vi "Write to IR DB.vi"(8 "error in (no error)":errorcluster, 9 "Values":u16[](array[numeric]), 10 "Modbus Address":u16, 11 "MB Cache in":refnum<class "MB Data Block.lvclass">) -> (0 "error out":errorcluster, 3 "MB Cache out":refnum<class "MB Data Block.lvclass">)   [LabVIEW 2018, in "MB PLC Client.lvlib" / "MB Data Block.lvclass"]
uses:
  MB Data Block.lvclass
  MB Data Block.lvclass/MB Data Block.ctl
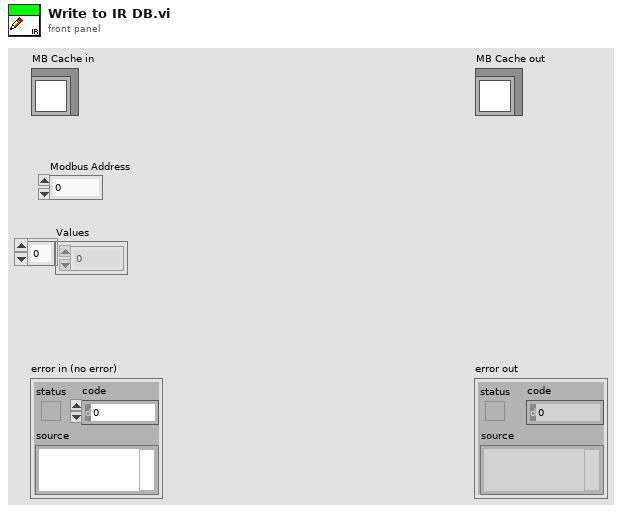
[diagram p1: front panel]
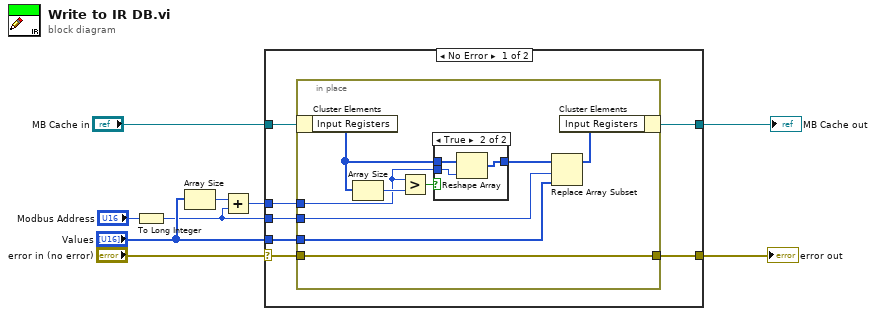
[diagram p0: block diagram]
diagram:
  n1 = To Long Integer(number="Modbus Address") -> (32bit integer=w5:i32)
  n2 = Array Size(array="Values") -> (size(s)=w6:i32)
  n3 = Add(x=w6, y=w5) -> (x+y=w4:i32)
  n4 = case shown="No Error" "error in (no error)" {
    selector: "error in (no error)" -> [w12 w31]
    tunnel: w4 -> [w16 _]
    tunnel: "Values" -> [w15 _]
    tunnel: [w11 w31] -> w2
    tunnel: w5 -> [w14 _]
    tunnel: "MB Cache in" -> [w13 w30]
    tunnel: [w10 w30] -> w1
    frame No Error {
      n5 = in-place {
        in-place-border: w16 -> [w23]
        in-place-border: w15 -> [w21]
        in-place-border: w14 -> [w18]
        in-place-border: [w17] -> w11
        in-place-border: w12 -> [w17]
        n6 = in-place-cluster #1(w13) -> ("Input Registers"=w20:u16[])
        n7 = Array Size(array=w20) -> (size(s)=w24:i32)
        n8 = Greater?(x=w23, y=w24) -> (0:w25:bool)
        n9 = case shown="True" w25 {
          tunnel: w20 -> [w26 w29]
          tunnel: [w26 w28] -> w22
          tunnel: w23 -> [_ w27]
          frame False {
          }
          frame True {
            n10 = Reshape Array(w29, w27) -> (w28:u16[])
          }
        }
        n11 = Replace Array Subset(array=w22, new element=w21, index=w18) -> (w19:u16[])
        n12 = in-place-cluster #1("Input Registers"=w19) -> (w10:refnum<class "MB Data Block.lvclass">)
      }
    }
    frame Error {
    }
  }
  "error out" <- w2
  "MB Cache out" <- w1
